vi "niDTS WLAN INSTR TX Configure PowerRamp.vi"(8 "error in (no error)":errorcluster, 11 "niDTS WLAN INSTR TX in":refnum<class "niDTS WLAN INSTR TX.lvclass">) -> (0 "error out":errorcluster, 3 "niDTS WLAN INSTR TX out":refnum<class "niDTS WLAN INSTR TX.lvclass">)   [LabVIEW 2015, in "niDTS WLAN.lvlib" / "niDTS WLAN INSTR TX.lvclass"]
doc: "Sets:\n\n* TxPowerEnabled\n* NumberOfAverages(txp)\n* MeasurementMode"
uses:
  niDTS WLAN INSTR TX.lvclass
  niDTS WLAN INSTR TX.lvclass/niDTS WLAN INSTR TX.ctl
  RiviInstDriver/niRfsaWlan/Objects/niRfsaWlan.lvclass
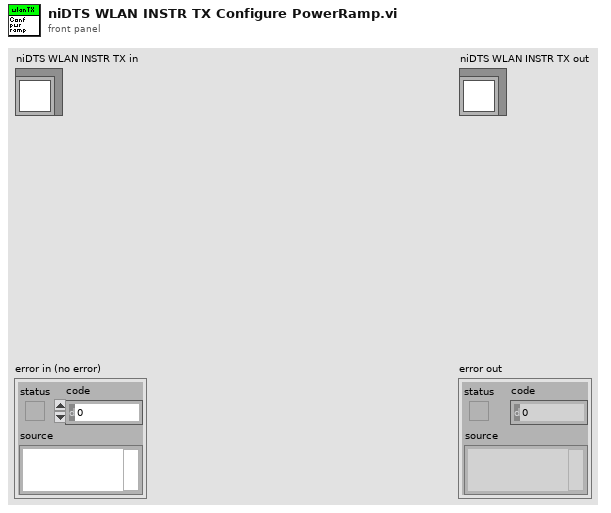
[diagram p1: front panel]
types:
  T1 = cluster{"RampUpLowThreshold":dbl, "RampUpHighThreshold":dbl, "RampDownLowThreshold":dbl, "RampDownHighThreshold":dbl}
  T2 = typedef "niDTS WLAN.lvlib/niDTS WLAN INC Standard.ctl" = enum16{"802.11 b DSSS", "802.11 a/g OFDM", "802.11 n HT", "802.11 ac VHT"}
  T3 = typedef "niRfsaWlan.lvclass/niRfsaWlan INC Handle.ctl" = refnum<data-value>
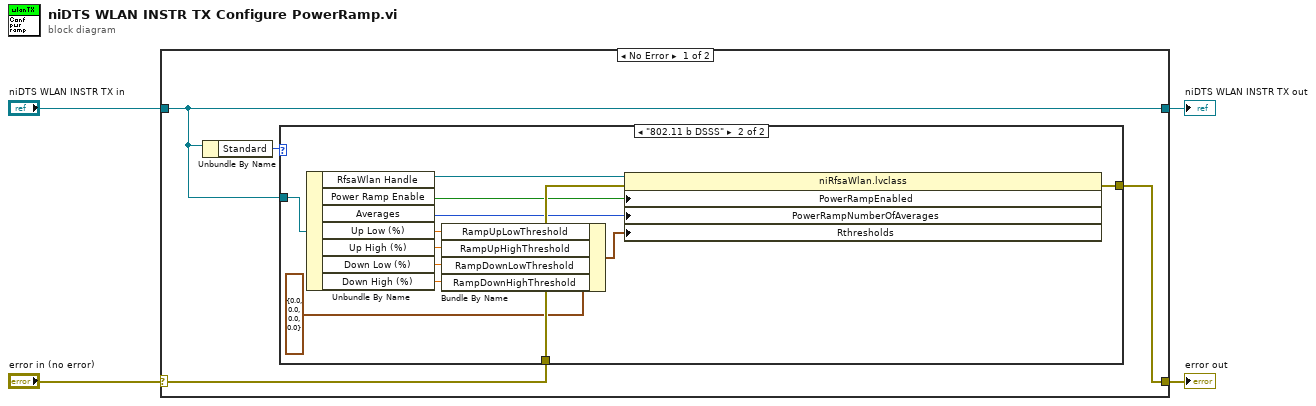
[diagram p0: block diagram]
diagram:
  n1 = case shown="No Error" "error in (no error)" {
    selector: "error in (no error)" -> [w8 w23]
    tunnel: [w7 w23] -> w3
    tunnel: [w6 w22] -> w1
    tunnel: "niDTS WLAN INSTR TX in" -> [w6 w22]
    frame No Error {
      n2 = Unbundle By Name(w6) -> ("Standard"=w5:T2)
      n3 = case shown="\"802.11 b DSSS\"" w5 {
        tunnel: w8 -> [w9 w20]
        tunnel: [w9 w19] -> w7
        tunnel: w6 -> [_ w18]
        frame Default {
        }
        frame "802.11 b DSSS" {
          n4 = Unbundle By Name(w18) -> ("RfsaWlan Handle"=w21:T3, "Power Ramp Enable"=w17:bool, "Averages"=w16:i32, "Up Low (%)"=w13:dbl, "Up High (%)"=w12:dbl, "Down Low (%)"=w11:dbl, "Down High (%)"=w10:dbl)
          n5 = Bundle By Name(cluster=T1 {"RampUpLowThreshold"=0.0, "RampUpHighThreshold"=0.0, "RampDownLowThreshold"=0.0, "RampDownHighThreshold"=0.0} ("CONFigure:RFSA:WLAN:MEASurement:PRAMp:RTHResholds"), "RampUpLowThreshold"=w13, "RampUpHighThreshold"=w12, "RampDownLowThreshold"=w11, "RampDownHighThreshold"=w10) -> (w14:T1)
          n6 = property class="niRfsaWlan.lvclass"(reference=w21, error in=w20, "PowerRampEnabled"=w17, "PowerRampNumberOfAverages"=w16, "Rthresholds"=w14) -> (error out=w19:errorcluster)  [unwired: 1 out]
        }
      }
    }
    frame Error {
    }
  }
  "error out" <- w3
  "niDTS WLAN INSTR TX out" <- w1
